vi "Variant to I32.vi"(10 "error in":errorcluster, 11 "data variant":variant) -> (2 "error out":errorcluster, 3 "data out":i32)   [LabVIEW 2018]
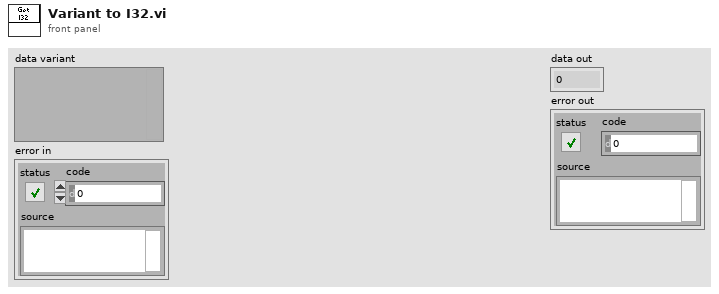
[diagram p1: front panel]
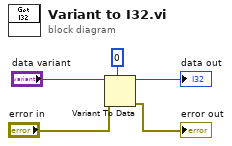
[diagram p0: block diagram]
diagram:
  n1 = Variant To Data(error in="error in", type=0, Variant="data variant") -> (data=→"data out":i32, error out=→"error out":errorcluster)
